vi "Running Max.vi"(3 "Starting Max":u32 caption="Starting Max (0)", 6 "Reset":bool caption="Reset (F)", 7 "Next Value":u32) -> (1 "Running Max":u32)   [LabVIEW 2016]
doc: "This SubVI keeps a running max value based on the input value and a starting max value. The current running max is resetable."
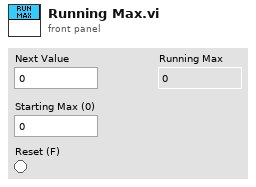
[diagram p1: front panel]
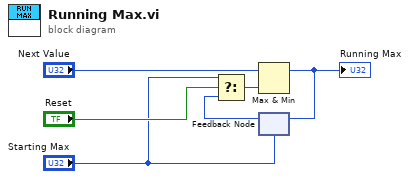
[diagram p0: block diagram]
diagram:
  n1 = feedback #1("Starting Max") -> (w3:u32)
  n2 = Select(t="Starting Max", s="Reset", f=w3) -> (s? t:f=w2:u32)
  n3 = Max & Min(x="Next Value", y=w2) -> (max(x,y)=w1:u32)  [unwired: 1 out]
  "Running Max" <- w1
  n4 = feedback-in #1(w1) -> ()
